vi "Configure.vi"(8 "error in (no error)":errorcluster caption="错误输入（无错误）", 10 "Function":T1=enum."AC Current", 11 "Keithley 2000 输入":refnum<class "Keithley 2000.lvclass">) -> (0 "error out":errorcluster caption="错误输出", 3 "Keithley 2000 输出":refnum<class "Keithley 2000.lvclass">)   [LabVIEW 2020, in "DMM.lvlib" / "Keithley 2000.lvclass"]
uses:
  Keithley 2000.lvclass
  D:/Workspace/LabVIEW/LVProject/Class/LVDevClass/DMM/root/DMM.lvclass
  root/Function.ctl
  <instrlib>/Keithley 2000/Public/Configure/Configure DC Volts.vi
  <instrlib>/Keithley 2000/Public/Configure/Configure DC Current.vi
  Keithley 2000.lvclass/Keithley 2000.ctl
  <instrlib>/Keithley 2000/Keithley 2000.lvlib
  root/DMM.lvclass
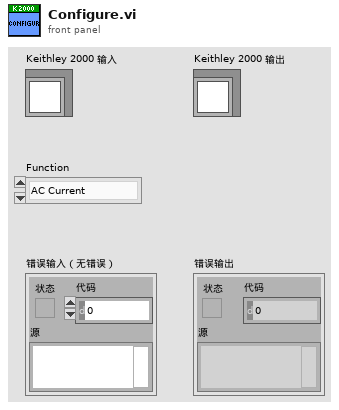
[diagram p1: front panel]
types:
  T1 = typedef "DMM.lvlib/DMM.lvclass/Function.ctl" = enum16{"DC Volts", "AC Volts", "DC Current", "AC Current", "2-Wire Resistance", "4-Wire Resistance"}
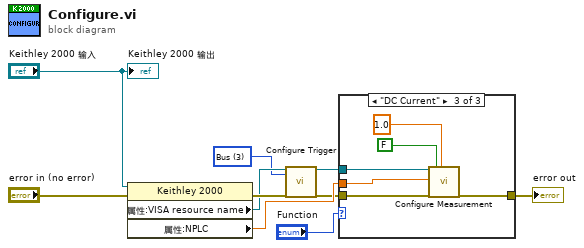
[diagram p0: block diagram]
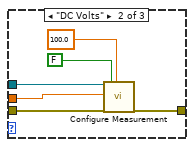
[diagram p3: hidden frame]
diagram:
  w1 = u16 3 items=["Immediate", "Timer", "Manual", "Bus", "External"] ("Source (0: Immediate)")
  n1 = property class="Keithley 2000"(reference="Keithley 2000 输入", error in="error in (no error)") -> (error out=w7:errorcluster, "属性:VISA resource name"=w3:refnum<visa-resource-name>, "属性:NPLC"=w5:dbl)  [unwired: 1 out]
  n2 = call <instrlib>:"Configure Trigger.vi"("VISA resource name"=w3, "Source (0: Immediate)"=w1, "error in (no error)"=w7) -> ("VISA resource name out"=w2:refnum<visa-resource-name>, "error out"=w4:errorcluster)  [unwired: 15 in]
  n3 = case shown="\"DC Current\"" "Function" {
    tunnel: w4 -> [w11 w17 w23]
    tunnel: w2 -> [_ w16 w22]
    tunnel: [w11 w15 w21] -> w6
    tunnel: w5 -> [_ w14 w20]
    frame Default {
    }
    frame "DC Volts" {
      n4 = call-poly <instrlib>:"Configure Measurement.vi"("VISA resource name"=w16, "Power Line Cycles (1.00)"=w14, "error in (no error)"=w17, "Auto Range? (T: Auto)"=FALSE, "Custom Range (0 V)"=100.0) -> ("error out"=w15:errorcluster)  [unwired: 13 in, 1 out]
    }
    frame "DC Current" {
      n5 = call-poly <instrlib>:"Configure Measurement.vi"("VISA resource name"=w22, "Power Line Cycles (1.00)"=w20, "error in (no error)"=w23, "Auto Range? (T: Auto)"=FALSE, "Custom Range (0 A)"=1.0) -> ("error out"=w21:errorcluster)  [unwired: 13 in, 1 out]
    }
  }
  "error out" <- w6
  "Keithley 2000 输出" <- "Keithley 2000 输入"
